vi "Rapid Read.vi"(0 "AlazarCluster":T10, 2 "Forward?":bool, 5 "Motion Settings":T2={"No Motion?"=FALSE, "Motion System"=enum."NI 735x", "Motion Bd ID"=1, "Motion Profile"="SMAC1", "# Axis"=1, "Reverse Z axis?"=TRUE, "SMAC Axis"=0, "scan pair"=enum."y-(x) scan", "RT fps"=6.0, "Steps per mm"=[1000, 1000, 1000, 1000], "Motor Parameters"={"velocity ct/s"=[10000.0, 10000.0, 10000.0, 50000.0], "accel ct/s^2"=[50000.0, 50000.0, 50000.0, 200000.0]}, "One Way Scan"=FALSE, "Reverse One Way Scan"=FALSE, "Global Position (mm)"=[], "Plane"=0, "Distance between\nscan lines (um)"=0.0, "Distance between\nscan planes (um)"=0.0, "number of scan planes"=1, "Total steps in line"=0, "Xtra plane\ndistance  (um)"=100, "Xtra planes "=1, "Add Axis"=FALSE, "overshoot cts"=200, "BKPT Shift"=0, "Scan Start Time (ms)"=0, "ESP VISA"="GPIB::1::INSTR", "3rd Axis"=1, "GL Ref Out"=refnum, "Galil Address"=""} {"3rd Axis" items=["x", "y", "z", "w"]; "Xtra planes" min=1; "Xtra plane\ndistance  (um)" min=0; "Distance between\nscan planes (um)" format="%.2f"; "Distance between\nscan lines (um)" format="%.2f"; "SMAC Axis" items=["None"=0, "Axis 1"=1, "Axis 2"=2, "Axis 3"=3, "Axis 4"=4, "Axis 5"=5, "Axis 6"=6, "Axis 7"=7, "Axis 8"=8, "Vector Space 1"=17, "Vector Space 2"=18, "Vector Space 3"=19, "Vector Space 4"=20]; "Motion Bd ID" min=1 max=32 step=1}, 7 "Digitizer Settings":T6={"Digitizer delay (us) "=0.0, "rf points per line"=2048, "lines per plane"=128, "Samp Rate (Hz)"=100000000.0, "Additional dig delay (us)"=0.0, "Voltage Scale"=0.4, "Pre-Looks"=0, "Offset delay (us)"=0.0, "bits A/D"=8, "Avg Num"=1, "DigTimeOut"=5.0, "Rel Dig Delay"=0.0, "Dig Ch"=0, "LeCroyCluster"={"LeCroy Channels"=[TRUE, FALSE, FALSE, FALSE], "LC read pt offset"=0.0, "Sweep Avg"=FALSE}, "Main Digitizer"=enum."NI Digitizer", "Dig Config"=enum."Single channel", "Digitizer ID Cluster"={"Acqiris/Alazar/SP ID"=[], "NI Instr Handles"=[], "LeCroy VISA"="", "GaGe Handle"={"Handle"=0, "Sample size"=0, "Resolution"=0, "Offset"=0, "Channels"=0, "Boards"=0}, "ATS Ref"="ATS9350", "Acqiris Address"=["PCI::INSTR0"], "ADQRef"=refnum, "adq_cu_ptr"=refnum}, "Trigger Settings"={"Trig Source"=1, "Trig Coupling"=0, "Trig Slope"=0, "Level (mV)"=1500.0}, "Bulk Acq"=FALSE, "Bulk Start Indexes"=[], "Data Ref RF"=refnum, "NI ID/Channel"=[], "Total Dig CH"=1, "Xtra Ann Trig delay (us)"=10.0, "Fix Z Delay?"=FALSE, "One Way Transmission?"=FALSE, "Data Ref Log"=refnum} {"Trigger Settings"."Trig Slope" items=["Positive", "Negative"]; "Trigger Settings"."Level (mV)" format="%.2f"; "Trigger Settings"."Trig Coupling" items=["DC 1 MOhm", "AC 1 MOhm", "DC 50 Ohm", "AC 50 Ohm"]; "Trigger Settings"."Trig Source" items=["Chan 1", "External"]; "Rel Dig Delay" format="%.2f"; "DigTimeOut" format="%.2f"; "Avg Num" min=1; "Offset delay (us)" format="%.2f"; "Additional dig delay (us)" format="%.2f"; "Digitizer delay (us)" format="%.2f"}, 9 "Location":T1=enum."WCM Main", 11 "error in":errorcluster, 12 "Pause?":bool, 13 "DigTimeOut":sgl=5.0 format="%.2f") -> (1 "gain":dbl, 4 "Array":i16[][](array[numeric]), 6 "Reverse?":bool, 8 "dig error":bool, 14 "gain 2 Ch":dbl, 15 "error out":errorcluster)   [LabVIEW 2022 SP3]
uses:
  -DigitizerRoutines/DigitizerSettings.ctl
  -DigitizerRoutines/Digitizer.ctl
  -DigitizerRoutines/DigConfig.ctl
  -DigitizerRoutines/DigitizerID.ctl
  C:/Windows/System32/ADQAPI_dotNet_helper.dll
  Windows/System32/ADQAPI_dotNet_helper.dll
  Motion Controllers/NI_controller/-NI_MotionRoutines/MotionParameters.ctl
  Motion Controllers/NI_controller/-NI_MotionRoutines/MotionSys.ctl
  Motion Controllers/-MotionRoutines/ScanAxis.ctl
  Motion Controllers/-MotionRoutines/3rdAxis.ctl
  -ScanSystem/Controls/location.ctl
  Motion Controllers/Galil/Command Menu.ctl
  <vilib>/DAQmx/write.llb/DAQmx Write (Digital Bool 1Line 1Point).vi
  Motion Controllers/-MotionRoutines/MotionGlobals.vi
  <vilib>/DAQmx/miscellaneous.llb/DAQmx Fill In Error Info.vi
  <instrlib>/niScope/Acquire/Fetch/niScope Multi Fetch Binary 8.vi
  <instrlib>/Acqiris Dx/Acqiris Dx.lvlib
  <vilib>/Motion/FlexMotion/CustomControls/CustomControls.llb/Program.flx
  <instrlib>/LeCroy Wave Series/LeCroy Wave Series.lvlib
panel:
  in  "Motion Program":u8=1 format="%.0x"
  # "1-D and 2-D B scan settings"
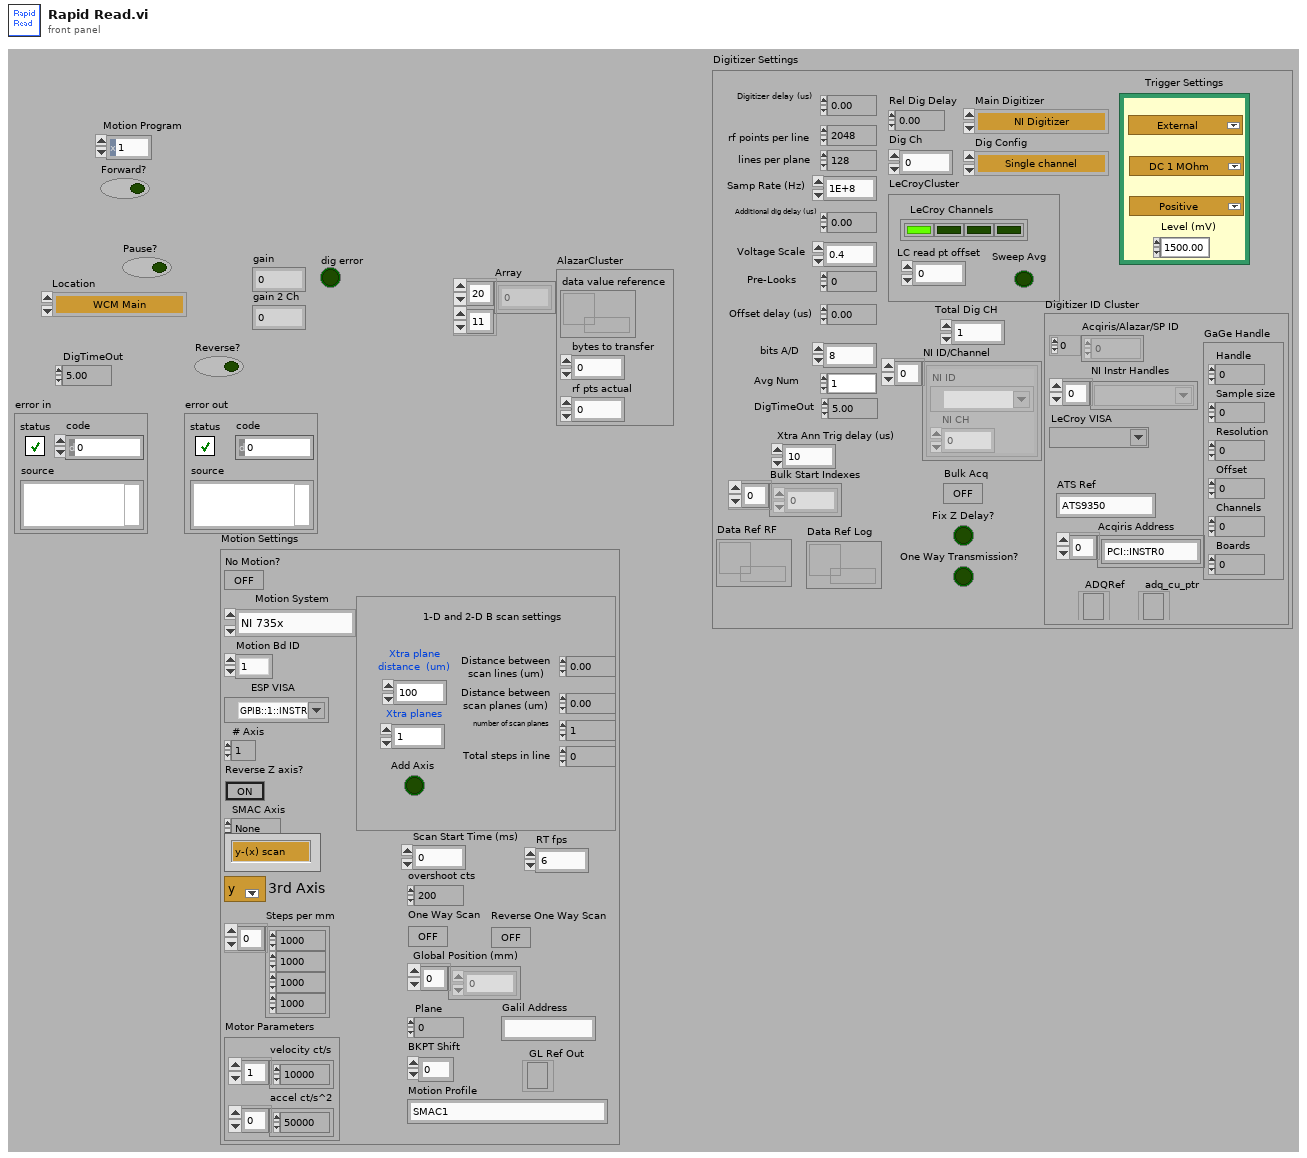
[diagram p1: front panel]
types:
  T1 = typedef "location.ctl" = enum16{"Automatic", "WCM Main", "Hawaii", "Columbia MM3000", "Columbia  NI System", "NYU", "RRI 2", "UHI Allen", "CUMC RT", "Chiba", "Stony Brook", "WCM Microscopy", "WCM Aeoretch", "WCM Optics Lab", "WCM Main 2Axis", "WCM Rotation", "WCM SAM SMAC", "SERI GP"}
  T2 = typedef "MotionParameters.ctl" = cluster{"No Motion?":bool, "Motion System":T3, "Motion Bd ID":u8, "Motion Profile":string, "# Axis":i8, "Reverse Z axis?":bool, "SMAC Axis":u16, "scan pair":T4, "RT fps":sgl, "Steps per mm":i32[], "Motor Parameters":cluster{"velocity ct/s":dbl[], "accel ct/s^2":dbl[]}, "One Way Scan":bool, "Reverse One Way Scan":bool, "Global Position (mm)":dbl[], "Plane":i32, "Distance between\nscan lines (um)":sgl, "Distance between\nscan planes (um)":sgl, "number of scan planes":i32, "Total steps in line":i32, "Xtra plane\ndistance  (um)":i32, "Xtra planes ":i32, "Add Axis":bool, "overshoot cts":i32, "BKPT Shift":i32, "Scan Start Time (ms)":u32, "ESP VISA":refnum<visa-resource-name>, "3rd Axis":T5, "GL Ref Out":refnum<k7>, "Galil Address":string}
  T3 = typedef "MotionSys.ctl" = enum16{"MM3000", "NI 735x", "Newport ESP", "No Motion Card", "Galil"}
  T4 = typedef "ScanAxis.ctl" = enum16{"y-(x) scan", "x-(y) scan", "z-(x) scan", "z-(y) scan", "y-(z) scan", "x-(z) scan", "w-(x) scan", "w-(y) scan", "w-(z) scan", "x-(w) scan", "y-(w) scan", "z-(w) scan"}
  T5 = typedef "3rdAxis.ctl" = u16
  T6 = typedef "DigitizerSettings.ctl" = cluster{"Digitizer delay (us) ":dbl, "rf points per line":i32, "lines per plane":i32, "Samp Rate (Hz)":dbl, "Additional dig delay (us)":dbl, "Voltage Scale":dbl, "Pre-Looks":i32, "Offset delay (us)":dbl, "bits A/D":i8, "Avg Num":i32, "DigTimeOut":sgl, "Rel Dig Delay":sgl, "Dig Ch":i32, "LeCroyCluster":cluster{"LeCroy Channels":bool[], "LC read pt offset":dbl, "Sweep Avg":bool}, "Main Digitizer":T7, "Dig Config":T8, "Digitizer ID Cluster":T9, "Trigger Settings":cluster{"Trig Source":u16, "Trig Coupling":u16, "Trig Slope":u16, "Level (mV)":dbl}, "Bulk Acq":bool, "Bulk Start Indexes":i32[], "Data Ref RF":refnum<data-value>, "NI ID/Channel":cluster{"NI ID":refnum<k15>, "NI CH":i32}[], "Total Dig CH":i32, "Xtra Ann Trig delay (us)":dbl, "Fix Z Delay?":bool, "One Way Transmission?":bool, "Data Ref Log":refnum<data-value>}
  T7 = typedef "Digitizer.ctl" = enum16{"Acqiris Digitizer", "NI Digitizer", "LeCroy", "GaGe", "AlazarTech", "No Digitizer", "Teledyne"}
  T8 = typedef "DigConfig.ctl" = enum16{"Single channel", "2 Chans w/ 2 Acqiris", "2 Chans w/ 1 Acqiris", "5-CH Pulser New", "5-CH pulser w/ ann array", "5-pass style ann array", "Empty"}
  T9 = typedef "DigitizerID.ctl" = cluster{"Acqiris/Alazar/SP ID":u32[], "NI Instr Handles":refnum<k15>[], "LeCroy VISA":refnum<visa-resource-name>, "GaGe Handle":cluster{"Handle":u32, "Sample size":u32, "Resolution":i32, "Offset":i32, "Channels":u32, "Boards":u32}, "ATS Ref":string, "Acqiris Address":string[], "ADQRef":refnum<k24>, "adq_cu_ptr":refnum<k24>}
  T10 = cluster{"data value reference":refnum<data-value>, "bytes to transfer":u32, "rf pts actual":u32}
  T11 = typedef "Command Menu.ctl" = enum16{"CommandPassThrough", "Abort Motion", "Define Pos", "Velocity", "Acceleration", "Deceleration", "Position Rel", "Postion Abs", "Begin Move", "After Move", "Home", "KI", "KD", "KP", "IL", "Config I/O", "Set Bit", "Clear Bit", "Motor Off", "Moto On", "Status", "Execute", "Halt Execute", "HX Status", "Tell Velocity", "Check Motion", "BreakPoint", "Tell Position", "Current Code Line", "Tell Switches", "OC Force On", "OC Off", "Pos Soft Limit", "Rev Soft Limit"}
  T12 = typedef "Program.flx" = u8
  T13 = typedef "Var" = u8
  T14 = typedef "Resource Out.flx" = u8
  T15 = cluster{"returnedSamplesPerSeg":i32, "indexFirstPoint":i32, "sampTime":dbl, "vGain":dbl, "vOffset":dbl, "returnedSegments":i32, "nbrAvgWforms":i32, "actualTriggersInAcqLo":u32, "actualTriggersInAcqHi":u32, "reserved3":dbl, "actualDataSize":u32, "missingValue":dbl}
  T16 = cluster{"actualSamples":i32, "absoluteInitialX":dbl, "relativeInitialX":dbl, "xIncrement":dbl, "offset":dbl, "gain":dbl, "reserved1":dbl, "reserved2":dbl}[]
  T17 = cluster{"actualSamples":i32, "absoluteInitialX":dbl, "relativeInitialX":dbl, "xIncrement":dbl, "offset":dbl, "gain":dbl, "reserved1":dbl, "reserved2":dbl}
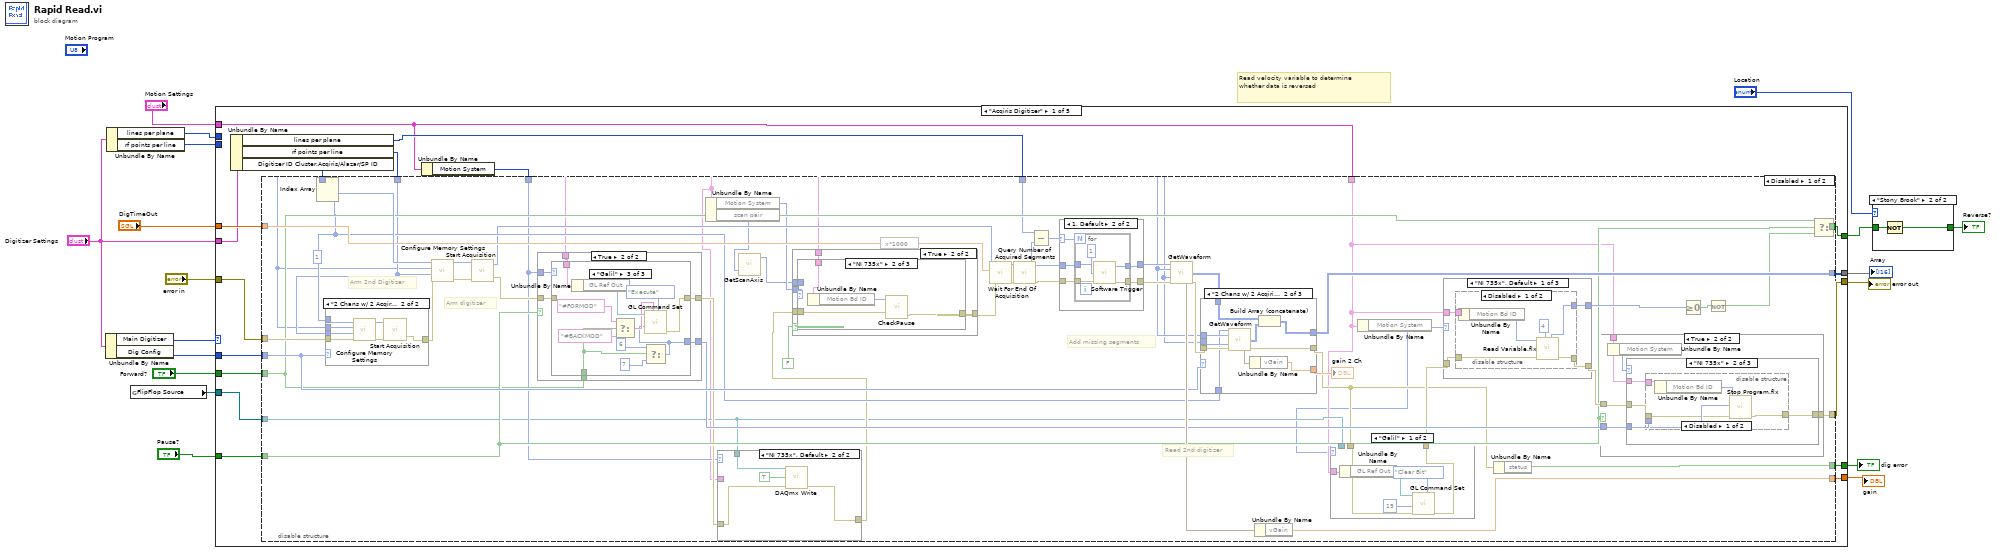
[diagram p0: block diagram]
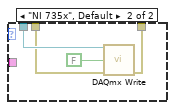
[diagram p3: hidden frame]
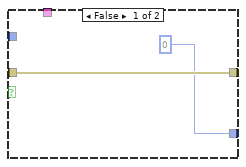
[diagram p4: hidden frame]
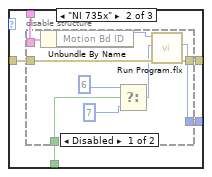
[diagram p6: hidden frame]
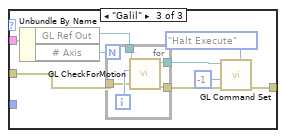
[diagram p11: hidden frame]
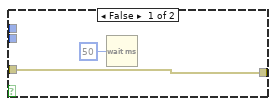
[diagram p12: hidden frame]
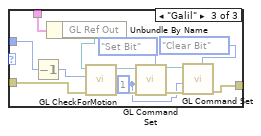
[diagram p14: hidden frame]
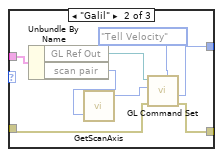
[diagram p16: hidden frame]
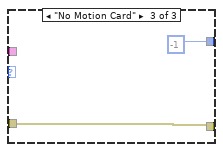
[diagram p17: hidden frame]
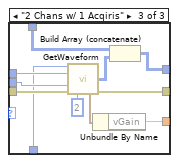
[diagram p19: hidden frame]
diagram:
  # "Read velocity variable to determine whether data is reversed"
  n1 = Unbundle By Name("Digitizer Settings") -> ("Main Digitizer"=w11:T7, "Dig Config"=w10:T8)
  n2 = Unbundle By Name("Digitizer Settings") -> ("lines per plane"=w8:i32, "rf points per line"=w7:i32)
  n3 = global read "MotionGlobals.vi" "FlipFlop Source"() -> (w14:refnum<k21>)
  n4 = case shown="\"Acqiris Digitizer\"" w11 {
    tunnel: [w26 w289 w441 w619 w763] -> w18
    tunnel: "error in" -> [w27 w284 w467 w614 w766]
    tunnel: w7 -> [_ _ _ _ _]
    tunnel: w8 -> [_ _ _ _ _]
    tunnel: [w35 w279 w459 w609 w789] -> w16
    tunnel: [w28 w295 w451 w626 w776] -> w5
    tunnel: "DigTimeOut" -> [w31 _ w458 _ w774]
    tunnel: [w34 w276 w461 w607 w785] -> w15
    tunnel: w14 -> [w20 w263 w432 w601 w762]
    tunnel: [w32 w297 w455 w629 w782] -> w13
    tunnel: "Digitizer Settings" -> [w30 w273 w445 w613 w768]
    tunnel: w10 -> [w29 _ _ _ _]
    tunnel: "Motion Settings" -> [w19 w259 w429 w599 w760]
    tunnel: "Pause?" -> [w25 w290 w442 w620 w773]
    tunnel: "Forward?" -> [w24 w291 w446 w622 _]
    frame "Acqiris Digitizer" {
      n5 = Unbundle By Name(w30) -> ("lines per plane"=w22:i32, "rf points per line"=w23:i32, "Digitizer ID Cluster.Acqiris/Alazar/SP ID"=w33:u32[])
      n6 = Unbundle By Name(w19) -> ("Motion System"=w21:T3)
      n7 = disable-structure shown="Disabled" {
        disable-tunnel: [w73 _] -> w35
        disable-tunnel: [w70 _] -> w34
        disable-tunnel: w33 -> [w67 _]
        disable-tunnel: [w66 _] -> w32
        disable-tunnel: w31 -> [w65 _]
        disable-tunnel: w29 -> [w63 _]
        disable-tunnel: [w61 _] -> w28
        disable-tunnel: w27 -> [w60 _]
        disable-tunnel: [w55 _] -> w26
        disable-tunnel: w25 -> [w53 _]
        disable-tunnel: w24 -> [w52 _]
        disable-tunnel: w23 -> [w45 _]
        disable-tunnel: w22 -> [w44 _]
        disable-tunnel: w21 -> [w41 _]
        disable-tunnel: w20 -> [w40 _]
        disable-tunnel: w19 -> [w37 _]
        frame Disabled {
          (unwired) 1 ("index")
          # "Read 2nd digitizer"
          # "Arm 2nd Digitizer"
          # "Arm digitizer"
          # "Add missing segments"
          n8 = Index Array(array=w67) -> (element #1=w68:u32, element #2=w50:u32)  [unwired: 2 in]
          n9 = case shown="\"2 Chans w/ 2 Acqiris\"" w63 {
            tunnel: w45 -> [_ w234]
            tunnel: w44 -> [_ w233]
            tunnel: w50 -> [_ w232]
            tunnel: w60 -> [w229 w231]
            tunnel: [w229 w230] -> w75
            frame "Single channel", Default {
            }
            frame "2 Chans w/ 2 Acqiris" {
              n10 = call <instrlib>:"Configure Memory Settings.vi"("error in (no error)"=w231, "Number of Samples (1000)"=w234, "Number of Segments (1)"=w233, "Instrument ID"=w232) -> ("error out"=w235:errorcluster, "dup Instrument ID"=w236:u32)  [unwired: 2 out]
              n11 = call <instrlib>:"Start Acquisition.vi"("error in (no error)"=w235, "Instrument ID"=w236) -> ("error out"=w230:errorcluster)  [unwired: 2 in, 1 out]
            }
          }
          n12 = call <instrlib>:"Configure Memory Settings.vi"("error in (no error)"=w75, "Number of Samples (1000)"=w45, "Number of Segments (1)"=w44, "Instrument ID"=w68) -> ("error out"=w78:errorcluster, "dup Instrument ID"=w79:u32)  [unwired: 2 out]
          n13 = call <instrlib>:"Start Acquisition.vi"("error in (no error)"=w78, "Instrument ID"=w79) -> ("error out"=w59:errorcluster, "dup Instrument ID"=w49:u32)  [unwired: 2 in]
          n14 = case shown="True" w53 {
            tunnel: w59 -> [w98 w104]
            tunnel: [w98 w103] -> w42
            tunnel: w52 -> [_ w102]
            tunnel: [u8 0 ("Resource Out") w101] -> w57
            tunnel: w41 -> [_ w100]
            tunnel: w37 -> [_ w99]
            frame False {
            }
            frame True {
              n15 = case shown="\"Galil\"" w100 {
                tunnel: w104 -> [w105 w110 _]
                tunnel: [w105 w109 w126] -> w103
                tunnel: w102 -> [_ w108 w122]
                tunnel: [_ w107 w120] -> w101
                tunnel: w99 -> [_ w106 w129]
                frame "MM3000", Default {
                }
                frame "NI 735x" {
                  n16 = disable-structure shown="Disabled" {
                    disable-tunnel: w110 -> [w119 _]
                    disable-tunnel: [w118 _] -> w109
                    disable-tunnel: w108 -> [w114 _]
                    disable-tunnel: [w113 _] -> w107
                    disable-tunnel: w106 -> [w112 _]
                    frame Disabled {
                      n17 = Unbundle By Name(w112) -> ("Motion Bd ID"=w111:u8)
                      n18 = Select(t=T12 6 ("Motion Program"), s=w114, f=T12 7 ("Motion Program")) -> (s? t:f=w115:T12)
                      n19 = call <vilib>:"Run Program.flx"("error in (no error)"=w119, "Program (1)"=w115, "Board ID"=w111) -> ("error out"=w118:errorcluster, "Resource Out"=w113:T14)  [unwired: 3 in, 1 out]
                    }
                    frame Enabled {
                    }
                  }
                }
                frame "Galil" {
                  n20 = Unbundle By Name(w129) -> ("GL Ref Out"=w128:refnum<k7>)
                  n21 = Select(t="#FORMOD" ("Program Name"), s=w122, f="#BACKMOD" ("Program Name")) -> (s? t:f=w127:string)
                  n22 = Select(t=u8 6 ("Motion Program"), s=w122, f=u8 7 ("Motion Program")) -> (s? t:f=w120:u8)
                  n23 = call "GL Command Set.vi"("Command"=Command_Menu."Execute", "Text Input"=w127, "Value"=w120, "Galil.IGalil"=w128) -> ("error out"=w126:errorcluster)  [unwired: 3 in, 4 out]
                }
              }
            }
          }
          n24 = Unbundle By Name(w37) -> ("Motion System"=w48:T3, "scan pair"=w47:T4)
          n25 = case shown="\"NI 735x\", Default" w41 {
            tunnel: w40 -> [_ w257]
            tunnel: w37 -> [w251 _]
            tunnel: w42 -> [w250 w256]
            tunnel: [w249 w255] -> w43
            frame "Galil" {
              n26 = Unbundle By Name(w251) -> ("GL Ref Out"=w254:refnum<k7>)
              n27 = call "GL Command Set.vi"("Command"=Command_Menu."Set Bit", "error in (no error)"=w250, "Value"=19, "Galil.IGalil"=w254) -> ("error out"=w249:errorcluster)  [unwired: 3 in, 4 out]
            }
            frame "NI 735x", Default {
              n28 = call-poly <vilib>:"DAQmx Write.vi"("task/channels in"=w257, "data"=TRUE ("stop (T)"), "error in"=w256) -> ("error out"=w255:errorcluster)  [unwired: 10 in, 2 out]
            }
          }
          n29 = call "GetScanAxis.vi"("scan pair"=w47) -> ("Axis 1"=w46:i32)  [unwired: 1 in, 2 out]
          n30 = case shown="True" FALSE {
            tunnel: w43 -> [w162 w167]
            tunnel: [w162 w166] -> w62
            tunnel: w37 -> [_ w165]
            tunnel: w48 -> [_ w164]
            tunnel: w46 -> [_ w163]
            frame False {
              n31 = Wait (ms)(milliseconds to wait=u32 50) -> ()  [unwired: 1 out]
            }
            frame True {
              n32 = case shown="\"NI 735x\"" w164 {
                tunnel: w167 -> [w168 w172 w179]
                tunnel: [w168 w171 w180] -> w166
                tunnel: w165 -> [_ w170 w178]
                tunnel: w163 -> [_ _ w176]
                frame "MM3000", Default {
                }
                frame "NI 735x" {
                  n33 = Unbundle By Name(w170) -> ("Motion Bd ID"=w169:u8)
                  n34 = call "CheckPause.vi"("error in"=w172, "Motion Board ID"=w169) -> ("error out"=w171:errorcluster)  [unwired: 3 in]
                }
                frame "Galil" {
                  w173 = 1 ("Value")
                  n35 = Decrement(x=w176) -> (x-1=w175:i32)
                  n36 = Unbundle By Name(w178) -> ("GL Ref Out"=w177:refnum<k7>)
                  n37 = call "GL CheckForMotion.vi"("error in"=w179, "Axis"=w175, "Refnum in"=w177) -> ("error out"=w184:errorcluster, "Refnum out"=w185:refnum<k7>)  [unwired: 6 in, 1 out]
                  n38 = call "GL Command Set.vi"("Command"=Command_Menu."Set Bit", "error in (no error)"=w184, "Value"=w173, "Galil.IGalil"=w185) -> ("error out"=w182:errorcluster, "ref out"=w181:refnum<k7>)  [unwired: 3 in, 3 out]
                  n39 = call "GL Command Set.vi"("Command"=Command_Menu."Clear Bit", "error in (no error)"=w182, "Value"=w173, "Galil.IGalil"=w181) -> ("error out"=w180:errorcluster)  [unwired: 3 in, 4 out]
                }
              }
            }
          }
          n40 = expression code="x*1000"(w65) -> (w64:sgl)
          n41 = call <instrlib>:"Wait For End Of Acquisition.vi"("error in (no error)"=w62, "Timeout"=w64, "Instrument ID"=w49) -> ("error out"=w77:errorcluster, "dup Instrument ID"=w83:u32)  [unwired: 3 out]
          n42 = call <instrlib>:"Query Number of Acquired Segments.vi"("error in (no error)"=w77, "Instrument ID"=w83) -> ("error out"=w85:errorcluster, "Number of Segments"=w86:i32, "dup Instrument ID"=w82:u32)  [unwired: 3 out]
          n43 = Subtract(x=w44, y=w86) -> (x-y=w81:i32)
          n44 = case shown="1, Default" w81 {
            selector: w81 -> [_ w239]
            tunnel: w85 -> [w237 w243]
            tunnel: [w237 w242] -> w84
            tunnel: w82 -> [w238 w241]
            tunnel: [w238 w240] -> w80
            frame 0 {
            }
            frame 1, Default {
              n45 = for {
                N: w239 -> [_]
                tunnel: w243 -> [w248]
                tunnel: w241 -> [w245]
                tunnel: [w247] -> w242
                tunnel: [w244] -> w240
                n46 = call <instrlib>:"Software Trigger.vi"("error in (no error)"=w248, "Type"=1, "Instrument ID"=w245) -> ("error out"=w247:errorcluster, "dup Instrument ID"=w244:u32)
              }
            }
          }
          n47 = call "GetWaveform.vi"("Acq ID Out"=w80, "Num Samps"=w45, "Num Segs"=w44, "error in"=w84) -> ("Acquired Waveform16 bit"=w72:i16[][], "dataDesc"=w71:T15, "error out"=w74:errorcluster)  [unwired: 2 in, 7 out]
          n48 = case shown="\"2 Chans w/ 2 Acqiris\"" w63 {
            tunnel: w74 -> [w207 w217 w228]
            tunnel: [w207 w216 w227] -> w38
            tunnel: w44 -> [_ w215 w226]
            tunnel: w45 -> [_ w214 w225]
            tunnel: w50 -> [_ w213 w224]
            tunnel: [w206 w210 w221] -> w73
            tunnel: w72 -> [w206 w212 w223]
            tunnel: [_ w208 w218] -> w69
            frame "Single channel", Default {
            }
            frame "2 Chans w/ 2 Acqiris" {
              n49 = call "GetWaveform.vi"("Acq ID Out"=w213, "Num Samps"=w214, "Num Segs"=w215, "error in"=w217) -> ("Acquired Waveform16 bit"=w211:i16[][], "dataDesc"=w209:T15, "error out"=w216:errorcluster)  [unwired: 2 in, 7 out]
              n50 = Unbundle By Name(w209) -> ("vGain"=w208:dbl)
              n51 = Build Array (concatenate)(w212, w211) -> (w210:i16[][])
            }
            frame "2 Chans w/ 1 Acqiris" {
              n52 = call "GetWaveform.vi"("Acq ID Out"=w224, "Num Samps"=w225, "Num Segs"=w226, "error in"=w228, "Channel"=2) -> ("Acquired Waveform16 bit"=w222:i16[][], "dataDesc"=w219:T15, "error out"=w227:errorcluster)  [unwired: 1 in, 7 out]
              n53 = Unbundle By Name(w219) -> ("vGain"=w218:dbl)
              n54 = Build Array (concatenate)(w223, w222) -> (w221:i16[][])
            }
          }
          "gain 2 Ch" <- w69
          n55 = Unbundle By Name(w71) -> ("vGain"=w70:dbl)
          n56 = Unbundle By Name(w37) -> ("Motion System"=w36:T3)
          n57 = case shown="\"Galil\"" w36 {
            tunnel: w40 -> [_ w95]
            tunnel: w37 -> [w89 _]
            tunnel: w38 -> [w88 w94]
            tunnel: [w87 w93] -> w39
            frame "Galil" {
              n58 = Unbundle By Name(w89) -> ("GL Ref Out"=w92:refnum<k7>)
              n59 = call "GL Command Set.vi"("Command"=Command_Menu."Clear Bit", "error in (no error)"=w88, "Value"=19, "Galil.IGalil"=w92) -> ("error out"=w87:errorcluster)  [unwired: 3 in, 4 out]
            }
            frame "NI 735x", Default {
              n60 = call-poly <vilib>:"DAQmx Write.vi"("task/channels in"=w95, "data"=FALSE ("stop (T)"), "error in"=w94) -> ("error out"=w93:errorcluster)  [unwired: 10 in, 2 out]
            }
          }
          n61 = case shown="\"NI 735x\", Default" w36 {
            tunnel: [w186 w197 -1 ("Output")] -> w76
            tunnel: [w189 w198 w204] -> w58
            tunnel: w39 -> [w188 w199 w204]
            tunnel: w37 -> [w187 w196 _]
            frame "NI 735x", Default {
              n62 = disable-structure shown="Disabled" {
                disable-tunnel: [w194 _] -> w189
                disable-tunnel: w188 -> [w193 _]
                disable-tunnel: w187 -> [w192 _]
                disable-tunnel: [w191 _] -> w186
                frame Disabled {
                  n63 = Unbundle By Name(w192) -> ("Motion Bd ID"=w190:u8)
                  n64 = call <vilib>:"Read Variable.flx"("Var"=T13 4, "error in (no error)"=w193, "Board ID"=w190) -> ("error out"=w194:errorcluster, "Output"=w191:i32)  [unwired: 1 in, 4 out]
                }
                frame Enabled {
                }
              }
            }
            frame "Galil" {
              n65 = Unbundle By Name(w196) -> ("GL Ref Out"=w202:refnum<k7>, "scan pair"=w201:T4)
              n66 = call "GetScanAxis.vi"("scan pair"=w201) -> ("Axis 1"=w200:i32)  [unwired: 1 in, 2 out]
              n67 = call "GL Command Set.vi"("Command"=Command_Menu."Tell Velocity", "error in (no error)"=w199, "Axis"=w200, "Galil.IGalil"=w202) -> ("error out"=w198:errorcluster, "Response#"=w197:i32)  [unwired: 3 in, 3 out]
            }
            frame "No Motion Card" {
            }
          }
          n68 = Unbundle By Name(w38) -> ("status"=w66:bool)
          n69 = case shown="True" w53 {
            tunnel: w57 -> [_ w135]
            tunnel: w58 -> [w131 w134]
            tunnel: [w131 w136] -> w55
            tunnel: w37 -> [_ w133]
            frame False {
            }
            frame True {
              n70 = Unbundle By Name(w133) -> ("Motion System"=w132:T3)
              n71 = case shown="\"NI 735x\"" w132 {
                tunnel: [w137 w141 w149] -> w136
                tunnel: w135 -> [_ w140 _]
                tunnel: w134 -> [w137 w138 w152]
                tunnel: w133 -> [_ w139 w153]
                frame "MM3000", Default {
                }
                frame "NI 735x" {
                  n72 = disable-structure shown="Disabled" {
                    disable-tunnel: [w146 _] -> w141
                    disable-tunnel: w140 -> [w145 _]
                    disable-tunnel: w139 -> [w143 _]
                    disable-tunnel: w138 -> [w142 _]
                    frame Disabled {
                      n73 = Unbundle By Name(w143) -> ("Motion Bd ID"=w144:u8)
                      n74 = call <vilib>:"Stop Program.flx"("error in (no error)"=w142, "Program (1)"=w145, "Board ID"=w144) -> ("error out"=w146:errorcluster)  [unwired: 3 in, 2 out]
                    }
                    frame Enabled {
                    }
                  }
                }
                frame "Galil" {
                  n75 = Unbundle By Name(w153) -> ("GL Ref Out"=w154:refnum<k7>, "# Axis"=w155:i8)
                  n76 = for {
                    N: w155 -> [_]
                    tunnel: [w160] -> w151
                    tunnel: w154 -> [w159]
                    tunnel: w152 -> [w157]
                    tunnel: [w156] -> w150
                    i -> [w158]
                    n77 = call "GL CheckForMotion.vi"("error in"=w157, "Axis"=w158, "Refnum in"=w159) -> ("error out"=w160:errorcluster, "Refnum out"=w156:refnum<k7>)  [unwired: 6 in, 1 out]
                  }
                  n78 = call "GL Command Set.vi"("Command"=Command_Menu."Halt Execute", "error in (no error)"=w151, "Value"=-1, "Galil.IGalil"=w150) -> ("error out"=w149:errorcluster)  [unwired: 3 in, 4 out]
                }
              }
            }
          }
          n79 = Greater Or Equal To 0?(x=w76) -> (x >= 0?=w54:bool)
          n80 = Not(x=w54) -> (.not. x?=w51:bool)
          n81 = Select(t=w52, s=w53, f=w51) -> (s? t:f=w61:bool)
        }
        frame Enabled {
        }
      }
    }
    frame "Teledyne" {
      # "Set flip flop to take next frame edge"
      # "Arm digitizer"
      n82 = Unbundle By Name(w273) -> ("Digitizer ID Cluster.ADQRef"=w283:refnum<k24>, "Digitizer ID Cluster.adq_cu_ptr"=w282:refnum<k24>, "Digitizer ID Cluster.GaGe Handle.Boards"=w281:u32)
      n83 = call "SPADQ_DisarmArmTrigger.vi"("error in (no error)"=w284, "adq_num"=w281, "adq_cu_ptr in"=w282, "ADQAPI Ref"=w283) -> ("error out"=w286:errorcluster, "ADQAPI Ref (out)"=w285:refnum<k24>)  [unwired: 6 in]
      n84 = call "SPADQ_ArmTrigger.vi"("error in (no error)"=w286, "adq_num"=w281, "adq_cu_ptr in"=w282, "ADQAPI Ref"=w285) -> ("error out"=w280:errorcluster)  [unwired: 6 in, 1 out]
      n85 = Unbundle By Name(w259) -> ("Motion System"=w266:T3)
      n86 = case shown="False" w290 {
        tunnel: w280 -> [w347 w353]
        tunnel: [w347 w352] -> w265
        tunnel: w291 -> [_ w351]
        tunnel: [u8 0 ("Resource Out") w350] -> w294
        tunnel: w266 -> [_ w349]
        tunnel: w259 -> [_ w348]
        frame False {
        }
        frame True {
          n87 = case shown="\"Galil\"" w349 {
            tunnel: w353 -> [w354 w359 _]
            tunnel: [w354 w358 w374] -> w352
            tunnel: w351 -> [_ w357 w370]
            tunnel: [_ w355 _] -> w350
            tunnel: w348 -> [_ w356 w373]
            frame "MM3000", Default {
            }
            frame "NI 735x" {
              n88 = disable-structure shown="Disabled" {
                disable-tunnel: w359 -> [w368 _]
                disable-tunnel: [w367 _] -> w358
                disable-tunnel: w357 -> [w363 _]
                disable-tunnel: w356 -> [w362 _]
                disable-tunnel: [w360 _] -> w355
                frame Disabled {
                  n89 = Unbundle By Name(w362) -> ("Motion Bd ID"=w361:u8)
                  n90 = Select(t=T12 6 ("Motion Program"), s=w363, f=T12 7 ("Motion Program")) -> (s? t:f=w364:T12)
                  n91 = call <vilib>:"Run Program.flx"("error in (no error)"=w368, "Program (1)"=w364, "Board ID"=w361) -> ("error out"=w367:errorcluster, "Resource Out"=w360:T14)  [unwired: 3 in, 1 out]
                }
                frame Enabled {
                }
              }
            }
            frame "Galil" {
              n92 = Unbundle By Name(w373) -> ("GL Ref Out"=w378:refnum<k7>)
              n93 = Select(t="#FORMOD" ("Program Name"), s=w370, f="#BACKMOD" ("Program Name")) -> (s? t:f=w377:string)
              n94 = Select(t=u8 6 ("Motion Program"), s=w370, f=u8 7 ("Motion Program")) -> (s? t:f=w371:u8)
              n95 = call "GL Command Set.vi"("Command"=Command_Menu."Execute", "Text Input"=w377, "Value"=w371, "Galil.IGalil"=w378) -> ("error out"=w374:errorcluster)  [unwired: 3 in, 4 out]
            }
          }
        }
      }
      n96 = case shown="\"NI 735x\", Default" w266 {
        tunnel: w263 -> [_ w316]
        tunnel: w265 -> [w310 w315]
        tunnel: [w309 w314] -> w264
        tunnel: w259 -> [w308 _]
        frame "Galil" {
          n97 = Unbundle By Name(w308) -> ("GL Ref Out"=w313:refnum<k7>)
          n98 = call "GL Command Set.vi"("Command"=Command_Menu."Set Bit", "error in (no error)"=w310, "Value"=19, "Galil.IGalil"=w313) -> ("error out"=w309:errorcluster)  [unwired: 3 in, 4 out]
        }
        frame "NI 735x", Default {
          n99 = call-poly <vilib>:"DAQmx Write.vi"("task/channels in"=w316, "data"=TRUE ("stop (T)"), "error in"=w315) -> ("error out"=w314:errorcluster)  [unwired: 10 in, 2 out]
        }
      }
      n100 = Unbundle By Name(w259) -> ("Motion System"=w260:T3)
      n101 = case shown="True" FALSE {
        tunnel: w264 -> [w381 w385]
        tunnel: [w381 w384] -> w287
        tunnel: w259 -> [_ w383]
        tunnel: w260 -> [_ w382]
        frame False {
          n102 = Wait (ms)(milliseconds to wait=u32 50) -> ()  [unwired: 1 out]
        }
        frame True {
          n103 = case shown="\"NI 735x\"" w382 {
            tunnel: w385 -> [w386 w390]
            tunnel: [w386 w389] -> w384
            tunnel: w383 -> [_ w388]
            frame "MM3000", Default {
            }
            frame "NI 735x" {
              n104 = Unbundle By Name(w388) -> ("Motion Bd ID"=w387:u8)
              n105 = call "CheckPause.vi"("error in"=w390, "Motion Board ID"=w387) -> ("error out"=w389:errorcluster)  [unwired: 3 in]
            }
          }
        }
      }
      n106 = case shown="\"NI 735x\", Default" w260 {
        tunnel: w287 -> [w411 w419 w427]
        tunnel: [w410 w419 w427] -> w274
        tunnel: [w409 -5 ("Output") w421] -> w288
        tunnel: w259 -> [w408 _ w426]
        frame "NI 735x", Default {
          n107 = disable-structure shown="Disabled" {
            disable-tunnel: w411 -> [w416 _]
            disable-tunnel: [w415 _] -> w410
            disable-tunnel: [w414 _] -> w409
            disable-tunnel: w408 -> [w413 _]
            frame Disabled {
              n108 = Unbundle By Name(w413) -> ("Motion Bd ID"=w412:u8)
              n109 = call <vilib>:"Read Variable.flx"("Var"=T13 4, "error in (no error)"=w416, "Board ID"=w412) -> ("error out"=w415:errorcluster, "Output"=w414:i32)  [unwired: 1 in, 4 out]
            }
            frame Enabled {
            }
          }
        }
        frame "No Motion Card" {
        }
        frame "Galil" {
          (unwired) -5 ("Output")
          n110 = Unbundle By Name(w426) -> ("GL Ref Out"=w425:refnum<k7>, "scan pair"=w423:T4)
          n111 = call "GetScanAxis.vi"("scan pair"=w423) -> ("Axis 1"=w422:i32)  [unwired: 1 in, 2 out]
          n112 = Decrement(x=w422) -> (x-1=w420:i32)
          n113 = call "GL Command Set.vi"("Command"=Command_Menu."Tell Velocity", "Axis"=w420, "Galil.IGalil"=w425) -> ("Response#"=w421:i32)  [unwired: 4 in, 4 out]
        }
      }
      n114 = Unbundle By Name(w273) -> ("Digitizer ID Cluster.ADQRef"=w272:refnum<k24>, "Digitizer ID Cluster.adq_cu_ptr"=w271:refnum<k24>, "Digitizer ID Cluster.GaGe Handle.Boards"=w270:u32, "DigTimeOut"=w269:sgl)
      n115 = Multiply(x=w269, y=sgl 1000.0) -> (x*y=w268:sgl)
      n116 = call "SPADQ_AcquisitionStatus.vi"("WaitTime (ms)"=w268, "error in (no error)"=w274, "adq_num"=w270, "adq_cu_ptr in"=w271, "ADQAPI Ref"=w272) -> ("error out"=w275:errorcluster)  [unwired: 3 in, 3 out]
      n117 = call "SPADQ_GetData.vi"("DelayCorrect?"=TRUE, "error in (no error)"=w275, "Digitizer Settings"=w273) -> ("error out"=w277:errorcluster, "Data Out"=w279:i16[][])  [unwired: 6 in, 1 out]
      n118 = case shown="\"NI 735x\", Default" w260 {
        tunnel: w277 -> [w393 w403 w407]
        tunnel: [w392 w402 w407] -> w262
        tunnel: w259 -> [w391 w405 _]
        frame "NI 735x", Default {
          n119 = disable-structure shown="Disabled" {
            disable-tunnel: w393 -> [w397 _]
            disable-tunnel: [w396 _] -> w392
            disable-tunnel: w391 -> [w395 _]
            frame Disabled {
              n120 = Unbundle By Name(w395) -> ("Motion Bd ID"=w394:u8)
              n121 = call <vilib>:"Read Variable.flx"("Var"=T13 4, "error in (no error)"=w397, "Board ID"=w394) -> ("error out"=w396:errorcluster)  [unwired: 1 in, 5 out]
            }
            frame Enabled {
            }
          }
        }
        frame "Galil" {
          n122 = Unbundle By Name(w405) -> ("GL Ref Out"=w404:refnum<k7>, "scan pair"=w401:T4)
          n123 = call "GetScanAxis.vi"("scan pair"=w401) -> ("Axis 1"=w400:i32)  [unwired: 1 in, 2 out]
          n124 = Decrement(x=w400) -> (x-1=w399:i32)
          n125 = call "GL Command Set.vi"("Command"=Command_Menu."Tell Velocity", "error in (no error)"=w403, "Axis"=w399, "Galil.IGalil"=w404) -> ("error out"=w402:errorcluster)  [unwired: 3 in, 4 out]
        }
        frame "No Motion Card" {
        }
      }
      n126 = call "Alazar_ConvertRaw.vi"("Digitizer Settings"=w273) -> ("Voltage multiplier"=w276:dbl)  [unwired: 9 in, 1 out]
      n127 = case shown="\"NI 735x\", Default" w260 {
        tunnel: w263 -> [_ w306]
        tunnel: w259 -> [w300 _]
        tunnel: w262 -> [w299 w305]
        tunnel: [w298 w304] -> w261
        frame "Galil" {
          n128 = Unbundle By Name(w300) -> ("GL Ref Out"=w303:refnum<k7>)
          n129 = call "GL Command Set.vi"("Command"=Command_Menu."Clear Bit", "error in (no error)"=w299, "Value"=19, "Galil.IGalil"=w303) -> ("error out"=w298:errorcluster)  [unwired: 3 in, 4 out]
        }
        frame "NI 735x", Default {
          n130 = call-poly <vilib>:"DAQmx Write.vi"("task/channels in"=w306, "data"=FALSE ("stop (T)"), "error in"=w305) -> ("error out"=w304:errorcluster)  [unwired: 10 in, 2 out]
        }
      }
      n131 = Less Than 0?(x=w288) -> (x < 0?=w296:bool)
      n132 = Not(x=w296) -> (.not. x?=w292:bool)
      n133 = case shown="False" w290 {
        tunnel: w294 -> [_ w323]
        tunnel: w261 -> [w318 w321]
        tunnel: [w318 w322] -> w289
        tunnel: w259 -> [_ w320]
        frame False {
        }
        frame True {
          n134 = Unbundle By Name(w320) -> ("Motion System"=w319:T3)
          n135 = case shown="\"NI 735x\"" w319 {
            tunnel: w323 -> [_ w328 _]
            tunnel: [w324 w327 w336] -> w322
            tunnel: w321 -> [w324 w326 w339]
            tunnel: w320 -> [_ w325 w341]
            frame "MM3000", Default {
            }
            frame "NI 735x" {
              n136 = disable-structure shown="Disabled" {
                disable-tunnel: w328 -> [w333 _]
                disable-tunnel: [w332 _] -> w327
                disable-tunnel: w326 -> [w331 _]
                disable-tunnel: w325 -> [w330 _]
                frame Disabled {
                  n137 = Unbundle By Name(w330) -> ("Motion Bd ID"=w329:u8)
                  n138 = call <vilib>:"Stop Program.flx"("error in (no error)"=w331, "Program (1)"=w333, "Board ID"=w329) -> ("error out"=w332:errorcluster)  [unwired: 3 in, 2 out]
                }
                frame Enabled {
                }
              }
            }
            frame "Galil" {
              n139 = Unbundle By Name(w341) -> ("GL Ref Out"=w335:refnum<k7>, "# Axis"=w340:i8)
              n140 = for {
                N: w340 -> [_]
                tunnel: [w345] -> w337
                tunnel: w335 -> [w344]
                tunnel: w339 -> [w342]
                i -> [w343]
                n141 = call "GL CheckForMotion.vi"("error in"=w342, "Axis"=w343, "Refnum in"=w344) -> ("error out"=w345:errorcluster)  [unwired: 6 in, 2 out]
              }
              n142 = call "GL Command Set.vi"("Command"=Command_Menu."Halt Execute", "error in (no error)"=w337, "Value"=-1, "Galil.IGalil"=w335) -> ("error out"=w336:errorcluster)  [unwired: 3 in, 4 out]
            }
          }
        }
      }
      n143 = Select(t=w292, s=w290, f=w291) -> (s? t:f=w295:bool)
      n144 = Unbundle By Name(w289) -> ("status"=w297:bool)
    }
    frame "NI Digitizer", Default {
      # "Set flip flop to take next frame edge"
      # "Arm digitizer"
      n145 = Unbundle By Name(w445) -> ("Digitizer ID Cluster.NI Instr Handles"=w457:refnum<k15>[])
      n146 = Index Array(array=w457) -> (element=w456:refnum<k15>)  [unwired: 1 in]
      n147 = call <instrlib>:"niScope Initiate Acquisition.vi"("instrument handle"=w456, "error in"=w467) -> ("instrument handle out"=w468:refnum<k15>, "error out"=w450:errorcluster)  [unwired: 1 in, 11 out]
      n148 = Unbundle By Name(w429) -> ("Motion System"=w444:T3)
      n149 = case shown="True" w442 {
        tunnel: w450 -> [w518 w524]
        tunnel: [w518 w523] -> w435
        tunnel: w446 -> [_ w522]
        tunnel: [u8 0 ("Resource Out") w521] -> w449
        tunnel: w444 -> [_ w520]
        tunnel: w429 -> [_ w519]
        frame False {
        }
        frame True {
          n150 = case shown="\"Galil\"" w520 {
            tunnel: w524 -> [w525 w530 _]
            tunnel: [w525 w529 w545] -> w523
            tunnel: w522 -> [_ w528 w541]
            tunnel: [_ w526 _] -> w521
            tunnel: w519 -> [_ w527 w544]
            frame "MM3000", Default {
            }
            frame "NI 735x" {
              n151 = disable-structure shown="Disabled" {
                disable-tunnel: w530 -> [w539 _]
                disable-tunnel: [w538 _] -> w529
                disable-tunnel: w528 -> [w534 _]
                disable-tunnel: w527 -> [w533 _]
                disable-tunnel: [w531 _] -> w526
                frame Disabled {
                  n152 = Unbundle By Name(w533) -> ("Motion Bd ID"=w532:u8)
                  n153 = Select(t=T12 6 ("Motion Program"), s=w534, f=T12 7 ("Motion Program")) -> (s? t:f=w535:T12)
                  n154 = call <vilib>:"Run Program.flx"("error in (no error)"=w539, "Program (1)"=w535, "Board ID"=w532) -> ("error out"=w538:errorcluster, "Resource Out"=w531:T14)  [unwired: 3 in, 1 out]
                }
                frame Enabled {
                }
              }
            }
            frame "Galil" {
              n155 = Unbundle By Name(w544) -> ("GL Ref Out"=w549:refnum<k7>)
              n156 = Select(t="#FORMOD" ("Program Name"), s=w541, f="#BACKMOD" ("Program Name")) -> (s? t:f=w548:string)
              n157 = Select(t=u8 6 ("Motion Program"), s=w541, f=u8 7 ("Motion Program")) -> (s? t:f=w542:u8)
              n158 = call "GL Command Set.vi"("Command"=Command_Menu."Execute", "Text Input"=w548, "Value"=w542, "Galil.IGalil"=w549) -> ("error out"=w545:errorcluster)  [unwired: 3 in, 4 out]
            }
          }
        }
      }
      n159 = Unbundle By Name(w429) -> ("Motion System"=w433:T3)
      n160 = case shown="\"NI 735x\", Default" w433 {
        tunnel: w432 -> [_ w487]
        tunnel: w429 -> [w481 _]
        tunnel: w435 -> [w480 w486]
        tunnel: [w479 w485] -> w434
        frame "Galil" {
          n161 = Unbundle By Name(w481) -> ("GL Ref Out"=w484:refnum<k7>)
          n162 = call "GL Command Set.vi"("Command"=Command_Menu."Set Bit", "error in (no error)"=w480, "Value"=19, "Galil.IGalil"=w484) -> ("error out"=w479:errorcluster)  [unwired: 3 in, 4 out]
        }
        frame "NI 735x", Default {
          n163 = call-poly <vilib>:"DAQmx Write.vi"("task/channels in"=w487, "data"=TRUE ("stop (T)"), "error in"=w486) -> ("error out"=w485:errorcluster)  [unwired: 10 in, 2 out]
        }
      }
      n164 = Unbundle By Name(w429) -> ("Motion System"=w443:T3)
      n165 = case shown="True" FALSE {
        tunnel: w434 -> [w552 w556]
        tunnel: [w552 w555] -> w439
        tunnel: w429 -> [_ w554]
        tunnel: w443 -> [_ w553]
        frame False {
          n166 = Wait (ms)(milliseconds to wait=u32 50) -> ()  [unwired: 1 out]
        }
        frame True {
          n167 = case shown="\"NI 735x\"" w553 {
            tunnel: w556 -> [w557 w561]
            tunnel: [w557 w560] -> w555
            tunnel: w554 -> [_ w559]
            frame "MM3000", Default {
            }
            frame "NI 735x" {
              n168 = Unbundle By Name(w559) -> ("Motion Bd ID"=w558:u8)
              n169 = call "CheckPause.vi"("error in"=w561, "Motion Board ID"=w558) -> ("error out"=w560:errorcluster)  [unwired: 3 in]
            }
          }
        }
      }
      n170 = Unbundle By Name(w445) -> ("rf points per line"=w436:i32, "Dig Ch"=w454:i32)
      n171 = case shown="\"NI 735x\", Default" w443 {
        tunnel: w439 -> [w582 w590 w598]
        tunnel: [w581 w590 w598] -> w438
        tunnel: [w580 -5 ("Output") w592] -> w440
        tunnel: w429 -> [w579 _ w597]
        frame "NI 735x", Default {
          n172 = disable-structure shown="Disabled" {
            disable-tunnel: w582 -> [w587 _]
            disable-tunnel: [w586 _] -> w581
            disable-tunnel: [w585 _] -> w580
            disable-tunnel: w579 -> [w584 _]
            frame Disabled {
              n173 = Unbundle By Name(w584) -> ("Motion Bd ID"=w583:u8)
              n174 = call <vilib>:"Read Variable.flx"("Var"=T13 4, "error in (no error)"=w587, "Board ID"=w583) -> ("error out"=w586:errorcluster, "Output"=w585:i32)  [unwired: 1 in, 4 out]
            }
            frame Enabled {
            }
          }
        }
        frame "No Motion Card" {
        }
        frame "Galil" {
          (unwired) -5 ("Output")
          n175 = Unbundle By Name(w597) -> ("GL Ref Out"=w596:refnum<k7>, "scan pair"=w594:T4)
          n176 = call "GetScanAxis.vi"("scan pair"=w594) -> ("Axis 1"=w593:i32)  [unwired: 1 in, 2 out]
          n177 = Decrement(x=w593) -> (x-1=w591:i32)
          n178 = call "GL Command Set.vi"("Command"=Command_Menu."Tell Velocity", "Axis"=w591, "Galil.IGalil"=w596) -> ("Response#"=w592:i32)  [unwired: 4 in, 4 out]
        }
      }
      n179 = Number To Decimal String(number=w454) -> (decimal integer string=w453:string)  [unwired: 1 in]
      n180 = property class="niScope"(reference=w468, error in=w438, "Fetch Record Number"=0, "Fetch Number of Records"=-1) -> (reference out=w464:refnum<k15>, error out=w437:errorcluster)
      n181 = call-poly <instrlib>:"niScope Fetch (poly).vi"("timeout"=w458, "error in"=w437, "numSamples"=w436, "channels"=w453, "instrument handle"=w464) -> ("error out"=w460:errorcluster, "wfm"=w459:i8[][], "wfm info"=w463:T16)  [unwired: 4 out]
      n182 = case shown="\"NI 735x\", Default" w443 {
        tunnel: w460 -> [w564 w574 w578]
        tunnel: [w563 w573 w578] -> w431
        tunnel: w429 -> [w562 w576 _]
        frame "NI 735x", Default {
          n183 = disable-structure shown="Disabled" {
            disable-tunnel: w564 -> [w568 _]
            disable-tunnel: [w567 _] -> w563
            disable-tunnel: w562 -> [w566 _]
            frame Disabled {
              n184 = Unbundle By Name(w566) -> ("Motion Bd ID"=w565:u8)
              n185 = call <vilib>:"Read Variable.flx"("Var"=T13 4, "error in (no error)"=w568, "Board ID"=w565) -> ("error out"=w567:errorcluster)  [unwired: 1 in, 5 out]
            }
            frame Enabled {
            }
          }
        }
        frame "Galil" {
          n186 = Unbundle By Name(w576) -> ("GL Ref Out"=w575:refnum<k7>, "scan pair"=w572:T4)
          n187 = call "GetScanAxis.vi"("scan pair"=w572) -> ("Axis 1"=w571:i32)  [unwired: 1 in, 2 out]
          n188 = Decrement(x=w571) -> (x-1=w570:i32)
          n189 = call "GL Command Set.vi"("Command"=Command_Menu."Tell Velocity", "error in (no error)"=w574, "Axis"=w570, "Galil.IGalil"=w575) -> ("error out"=w573:errorcluster)  [unwired: 3 in, 4 out]
        }
        frame "No Motion Card" {
        }
      }
      n190 = Unbundle By Name(w429) -> ("Motion System"=w428:T3)
      n191 = case shown="\"NI 735x\", Default" w428 {
        tunnel: w432 -> [_ w477]
        tunnel: w429 -> [w471 _]
        tunnel: w431 -> [w470 w476]
        tunnel: [w469 w475] -> w430
        frame "Galil" {
          n192 = Unbundle By Name(w471) -> ("GL Ref Out"=w474:refnum<k7>)
          n193 = call "GL Command Set.vi"("Command"=Command_Menu."Clear Bit", "error in (no error)"=w470, "Value"=19, "Galil.IGalil"=w474) -> ("error out"=w469:errorcluster)  [unwired: 3 in, 4 out]
        }
        frame "NI 735x", Default {
          n194 = call-poly <vilib>:"DAQmx Write.vi"("task/channels in"=w477, "data"=FALSE ("stop (T)"), "error in"=w476) -> ("error out"=w475:errorcluster)  [unwired: 10 in, 2 out]
        }
      }
      n195 = Less Than 0?(x=w440) -> (x < 0?=w452:bool)
      n196 = Not(x=w452) -> (.not. x?=w447:bool)
      n197 = Select(t=w447, s=w442, f=w446) -> (s? t:f=w451:bool)
      n198 = case shown="True" w442 {
        tunnel: w449 -> [_ w494]
        tunnel: w430 -> [w489 w492]
        tunnel: [w489 w493] -> w441
        tunnel: w429 -> [_ w491]
        frame False {
        }
        frame True {
          n199 = Unbundle By Name(w491) -> ("Motion System"=w490:T3)
          n200 = case shown="\"NI 735x\"" w490 {
            tunnel: w494 -> [_ w499 _]
            tunnel: [w495 w498 w507] -> w493
            tunnel: w492 -> [w495 w497 w510]
            tunnel: w491 -> [_ w496 w512]
            frame "MM3000", Default {
            }
            frame "NI 735x" {
              n201 = disable-structure shown="Disabled" {
                disable-tunnel: w499 -> [w504 _]
                disable-tunnel: [w503 _] -> w498
                disable-tunnel: w497 -> [w502 _]
                disable-tunnel: w496 -> [w501 _]
                frame Disabled {
                  n202 = Unbundle By Name(w501) -> ("Motion Bd ID"=w500:u8)
                  n203 = call <vilib>:"Stop Program.flx"("error in (no error)"=w502, "Program (1)"=w504, "Board ID"=w500) -> ("error out"=w503:errorcluster)  [unwired: 3 in, 2 out]
                }
                frame Enabled {
                }
              }
            }
            frame "Galil" {
              n204 = Unbundle By Name(w512) -> ("GL Ref Out"=w506:refnum<k7>, "# Axis"=w511:i8)
              n205 = for {
                N: w511 -> [_]
                tunnel: [w516] -> w508
                tunnel: w506 -> [w515]
                tunnel: w510 -> [w513]
                i -> [w514]
                n206 = call "GL CheckForMotion.vi"("error in"=w513, "Axis"=w514, "Refnum in"=w515) -> ("error out"=w516:errorcluster)  [unwired: 6 in, 2 out]
              }
              n207 = call "GL Command Set.vi"("Command"=Command_Menu."Halt Execute", "error in (no error)"=w508, "Value"=-1, "Galil.IGalil"=w506) -> ("error out"=w507:errorcluster)  [unwired: 3 in, 4 out]
            }
          }
        }
      }
      n208 = Index Array(array=w463) -> (element=w462:T17)  [unwired: 1 in]
      n209 = Unbundle By Name(w441) -> ("status"=w455:bool)
      n210 = Unbundle By Name(w462) -> ("gain"=w461:dbl)
    }
    frame "LeCroy" {
      w611 = u16 0 items=["Channel 1", "Channel 2", "Channel 3", "Channel 4", "Memory 1", "Memory 2", "Memory 3", "Memory 4", "Function 1", "Function 2", "Function 3", "Function 4", "Function 5", "Function 6", "Function 7", "Function 8", "Other"] ("Source (0: Channel 1)")
      # "Set flip flop to take next frame edge"
      # "Arm digitizer"
      n211 = Unbundle By Name(w613) -> ("Digitizer ID Cluster.LeCroy VISA"=w615:refnum<visa-resource-name>)
      n212 = call <instrlib>:"Initiate.vi"("error in (no error)"=w614, "VISA resource name"=w615) -> ("error out"=w616:errorcluster)  [unwired: 8 in, 1 out]
      n213 = Unbundle By Name(w599) -> ("Motion System"=w621:T3)
      n214 = case shown="True" w620 {
        tunnel: w616 -> [w679 w685]
        tunnel: [w679 w684] -> w603
        tunnel: w622 -> [_ w683]
        tunnel: [u8 0 ("Resource Out") w682] -> w625
        tunnel: w621 -> [_ w681]
        tunnel: w599 -> [_ w680]
        frame False {
        }
        frame True {
          n215 = case shown="\"Galil\"" w681 {
            tunnel: w685 -> [w686 w691 _]
            tunnel: [w686 w690 w706] -> w684
            tunnel: w683 -> [_ w689 w702]
            tunnel: [_ w687 _] -> w682
            tunnel: w680 -> [_ w688 w705]
            frame "MM3000", Default {
            }
            frame "NI 735x" {
              n216 = disable-structure shown="Disabled" {
                disable-tunnel: w691 -> [w700 _]
                disable-tunnel: [w699 _] -> w690
                disable-tunnel: w689 -> [w695 _]
                disable-tunnel: w688 -> [w694 _]
                disable-tunnel: [w692 _] -> w687
                frame Disabled {
                  n217 = Unbundle By Name(w694) -> ("Motion Bd ID"=w693:u8)
                  n218 = Select(t=T12 6 ("Motion Program"), s=w695, f=T12 7 ("Motion Program")) -> (s? t:f=w696:T12)
                  n219 = call <vilib>:"Run Program.flx"("error in (no error)"=w700, "Program (1)"=w696, "Board ID"=w693) -> ("error out"=w699:errorcluster, "Resource Out"=w692:T14)  [unwired: 3 in, 1 out]
                }
                frame Enabled {
                }
              }
            }
            frame "Galil" {
              n220 = Unbundle By Name(w705) -> ("GL Ref Out"=w710:refnum<k7>)
              n221 = Select(t="#FORMOD" ("Program Name"), s=w702, f="#BACKMOD" ("Program Name")) -> (s? t:f=w709:string)
              n222 = Select(t=u8 6 ("Motion Program"), s=w702, f=u8 7 ("Motion Program")) -> (s? t:f=w703:u8)
              n223 = call "GL Command Set.vi"("Command"=Command_Menu."Execute", "Text Input"=w709, "Value"=w703, "Galil.IGalil"=w710) -> ("error out"=w706:errorcluster)  [unwired: 3 in, 4 out]
            }
          }
        }
      }
      n224 = Unbundle By Name(w599) -> ("Motion System"=w600:T3)
      n225 = case shown="\"Galil\"" w600 {
        tunnel: w601 -> [_ w638]
        tunnel: w599 -> [w632 _]
        tunnel: w603 -> [w631 w637]
        tunnel: [w630 w636] -> w602
        frame "Galil" {
          n226 = Unbundle By Name(w632) -> ("GL Ref Out"=w635:refnum<k7>)
          n227 = call "GL Command Set.vi"("Command"=Command_Menu."Set Bit", "error in (no error)"=w631, "Value"=19, "Galil.IGalil"=w635) -> ("error out"=w630:errorcluster)  [unwired: 3 in, 4 out]
        }
        frame "NI 735x", Default {
          n228 = call-poly <vilib>:"DAQmx Write.vi"("task/channels in"=w638, "data"=TRUE ("stop (T)"), "error in"=w637) -> ("error out"=w636:errorcluster)  [unwired: 10 in, 2 out]
        }
      }
      n229 = Unbundle By Name(w599) -> ("Motion System"=w604:T3)
      n230 = case shown="True" FALSE {
        tunnel: w602 -> [w713 w717]
        tunnel: [w713 w716] -> w617
        tunnel: w599 -> [_ w715]
        tunnel: w604 -> [_ w714]
        frame False {
          n231 = Wait (ms)(milliseconds to wait=u32 50) -> ()  [unwired: 1 out]
        }
        frame True {
          n232 = case shown="\"NI 735x\"" w714 {
            tunnel: w717 -> [w718 w722]
            tunnel: [w718 w721] -> w716
            tunnel: w715 -> [_ w720]
            frame "MM3000", Default {
            }
            frame "NI 735x" {
              n233 = Unbundle By Name(w720) -> ("Motion Bd ID"=w719:u8)
              n234 = call "CheckPause.vi"("error in"=w722, "Motion Board ID"=w719) -> ("error out"=w721:errorcluster)  [unwired: 3 in]
            }
          }
        }
      }
      n235 = Unbundle By Name(w613) -> ("Dig Ch"=w628:i32)  [unwired: 1 out]
      n236 = case shown="\"NI 735x\", Default" w604 {
        tunnel: w617 -> [w743 w751 w759]
        tunnel: [w742 w751 w759] -> w610
        tunnel: [w741 -5 ("Output") w753] -> w618
        tunnel: w599 -> [w740 _ w758]
        frame "NI 735x", Default {
          n237 = disable-structure shown="Disabled" {
            disable-tunnel: w743 -> [w748 _]
            disable-tunnel: [w747 _] -> w742
            disable-tunnel: [w746 _] -> w741
            disable-tunnel: w740 -> [w745 _]
            frame Disabled {
              n238 = Unbundle By Name(w745) -> ("Motion Bd ID"=w744:u8)
              n239 = call <vilib>:"Read Variable.flx"("Var"=T13 4, "error in (no error)"=w748, "Board ID"=w744) -> ("error out"=w747:errorcluster, "Output"=w746:i32)  [unwired: 1 in, 4 out]
            }
            frame Enabled {
            }
          }
        }
        frame "No Motion Card" {
        }
        frame "Galil" {
          (unwired) -5 ("Output")
          n240 = Unbundle By Name(w758) -> ("GL Ref Out"=w757:refnum<k7>, "scan pair"=w755:T4)
          n241 = call "GetScanAxis.vi"("scan pair"=w755) -> ("Axis 1"=w754:i32)  [unwired: 1 in, 2 out]
          n242 = Decrement(x=w754) -> (x-1=w752:i32)
          n243 = call "GL Command Set.vi"("Command"=Command_Menu."Tell Velocity", "Axis"=w752, "Galil.IGalil"=w757) -> ("Response#"=w753:i32)  [unwired: 4 in, 4 out]
        }
      }
      n244 = Number To Decimal String(number=w628) -> ()  [unwired: 1 in, 1 out]
      n245 = call "GetAcqSeqLeCroy.vi"("Digitizer Settings"=w613, "errorin"=w610, "Source (0: Channel 1)"=w611, "save?"=FALSE) -> ("Raw VGain (scale)"=w607:dbl, "Data Array"=w609:i16[][], "error out"=w608:errorcluster)  [unwired: 17 in, 4 out]
      n246 = case shown="\"NI 735x\", Default" w604 {
        tunnel: w608 -> [w725 w735 w739]
        tunnel: [w724 w734 w739] -> w605
        tunnel: w599 -> [w723 w737 _]
        frame "NI 735x", Default {
          n247 = disable-structure shown="Disabled" {
            disable-tunnel: w725 -> [w729 _]
            disable-tunnel: [w728 _] -> w724
            disable-tunnel: w723 -> [w727 _]
            frame Disabled {
              n248 = Unbundle By Name(w727) -> ("Motion Bd ID"=w726:u8)
              n249 = call <vilib>:"Read Variable.flx"("Var"=T13 4, "error in (no error)"=w729, "Board ID"=w726) -> ("error out"=w728:errorcluster)  [unwired: 1 in, 5 out]
            }
            frame Enabled {
            }
          }
        }
        frame "Galil" {
          n250 = Unbundle By Name(w737) -> ("GL Ref Out"=w736:refnum<k7>, "scan pair"=w733:T4)
          n251 = call "GetScanAxis.vi"("scan pair"=w733) -> ("Axis 1"=w732:i32)  [unwired: 1 in, 2 out]
          n252 = Decrement(x=w732) -> (x-1=w731:i32)
          n253 = call "GL Command Set.vi"("Command"=Command_Menu."Tell Velocity", "error in (no error)"=w735, "Axis"=w731, "Galil.IGalil"=w736) -> ("error out"=w734:errorcluster)  [unwired: 3 in, 4 out]
        }
        frame "No Motion Card" {
        }
      }
      n254 = case shown="\"NI 735x\", Default" w604 {
        tunnel: w601 -> [_ w648]
        tunnel: w599 -> [w640 _]
        tunnel: w605 -> [w642 w647]
        tunnel: [w641 w646] -> w606
        frame "Galil" {
          n255 = Unbundle By Name(w640) -> ("GL Ref Out"=w645:refnum<k7>)
          n256 = call "GL Command Set.vi"("Command"=Command_Menu."Clear Bit", "error in (no error)"=w642, "Value"=19, "Galil.IGalil"=w645) -> ("error out"=w641:errorcluster)  [unwired: 3 in, 4 out]
        }
        frame "NI 735x", Default {
          n257 = call-poly <vilib>:"DAQmx Write.vi"("task/channels in"=w648, "data"=FALSE ("stop (T)"), "error in"=w647) -> ("error out"=w646:errorcluster)  [unwired: 10 in, 2 out]
        }
      }
      n258 = Less Than 0?(x=w618) -> (x < 0?=w627:bool)
      n259 = Not(x=w627) -> (.not. x?=w623:bool)
      n260 = case shown="True" w620 {
        tunnel: w625 -> [_ w655]
        tunnel: w606 -> [w650 w653]
        tunnel: [w650 w654] -> w619
        tunnel: w599 -> [_ w652]
        frame False {
        }
        frame True {
          n261 = Unbundle By Name(w652) -> ("Motion System"=w651:T3)
          n262 = case shown="\"NI 735x\"" w651 {
            tunnel: w655 -> [_ w660 _]
            tunnel: [w656 w659 w668] -> w654
            tunnel: w653 -> [w656 w658 w671]
            tunnel: w652 -> [_ w657 w673]
            frame "MM3000", Default {
            }
            frame "NI 735x" {
              n263 = disable-structure shown="Disabled" {
                disable-tunnel: w660 -> [w665 _]
                disable-tunnel: [w664 _] -> w659
                disable-tunnel: w658 -> [w663 _]
                disable-tunnel: w657 -> [w662 _]
                frame Disabled {
                  n264 = Unbundle By Name(w662) -> ("Motion Bd ID"=w661:u8)
                  n265 = call <vilib>:"Stop Program.flx"("error in (no error)"=w663, "Program (1)"=w665, "Board ID"=w661) -> ("error out"=w664:errorcluster)  [unwired: 3 in, 2 out]
                }
                frame Enabled {
                }
              }
            }
            frame "Galil" {
              n266 = Unbundle By Name(w673) -> ("GL Ref Out"=w667:refnum<k7>, "# Axis"=w672:i8)
              n267 = for {
                N: w672 -> [_]
                tunnel: [w677] -> w669
                tunnel: w667 -> [w676]
                tunnel: w671 -> [w674]
                i -> [w675]
                n268 = call "GL CheckForMotion.vi"("error in"=w674, "Axis"=w675, "Refnum in"=w676) -> ("error out"=w677:errorcluster)  [unwired: 6 in, 2 out]
              }
              n269 = call "GL Command Set.vi"("Command"=Command_Menu."Halt Execute", "error in (no error)"=w669, "Value"=-1, "Galil.IGalil"=w667) -> ("error out"=w668:errorcluster)  [unwired: 3 in, 4 out]
            }
          }
        }
      }
      n270 = Select(t=w623, s=w620, f=w622) -> (s? t:f=w626:bool)
      n271 = Unbundle By Name(w619) -> ("status"=w629:bool)
    }
    frame "AlazarTech" {
      # "Set flip flop to take next frame edge"
      n272 = Unbundle By Name(w760) -> ("Motion System"=w765:T3)
      n273 = Unbundle By Name(w768) -> ("Digitizer ID Cluster.Acqiris/Alazar/SP ID"=w786:u32[])
      n274 = case shown="\"NI 735x\", Default" w765 {
        tunnel: w762 -> [_ w809]
        tunnel: w760 -> [w803 _]
        tunnel: w766 -> [w802 w807]
        tunnel: [w801 w808] -> w767
        frame "Galil" {
          n275 = Unbundle By Name(w803) -> ("GL Ref Out"=w806:refnum<k7>)
          n276 = call "GL Command Set.vi"("Command"=Command_Menu."Set Bit", "error in (no error)"=w802, "Value"=19, "Galil.IGalil"=w806) -> ("error out"=w801:errorcluster)  [unwired: 3 in, 4 out]
        }
        frame "NI 735x", Default {
          n277 = call-poly <vilib>:"DAQmx Write.vi"("task/channels in"=w809, "data"=TRUE ("stop (T)"), "error in"=w807) -> ("error out"=w808:errorcluster)  [unwired: 10 in, 2 out]
        }
      }
      n278 = Index Array(array=w786) -> (element=w779:u32)  [unwired: 1 in]
      n279 = call "Rapid Read_Alazar_Done - ATS-SDK.vi"("Handle"=w779, "Motion Settings"=w760, "error out"=w767, "Pause?"=w773) -> ("Handle Out"=w778:u32, "Reverse?"=w776:bool, "error out"=w775:errorcluster)  [unwired: 9 in]
      n280 = case shown="14" 0 ("lines per plane") {
        tunnel: [_ u16 3 ("Extra Shift")] -> w781
        frame 0, Default {
        }
        frame 14 {
        }
      }
      n281 = expression code="x*1000"(w774) -> (w780:sgl)
      n282 = Unbundle By Name(w768) -> ("lines per plane"=w770:i32, "rf points per line"=w769:i32)
      n283 = call "AlazarReadBuffer - ATS-SDK.vi"("Handle"=w778, "Digitizer Settings"=w768, "time out (ms)"=w780, "AlazarCluster"="AlazarCluster", "Extra Shift"=w781, "error in (no error)"=w775) -> ("Data Array"=w772:i16[], "Return Code"=w783:u32, "Voltage Scale"=w785:dbl, "error out"=w764:errorcluster)  [unwired: 5 in, 1 out]
      n284 = Unbundle By Name("AlazarCluster") -> ("rf pts actual"=w790:u32)
      n285 = Equal?(x=w783, y=u32 579) -> (x = y?=w782:bool)
      n286 = call "DelayPtsAdjust.vi"("Digitizer Settings"=w768) -> ("PostDelayCorrection"=w771:u32)  [unwired: 9 in, 1 out]
      n287 = Reshape Array(w772, w770, w790) -> (w788:i16[][])
      n288 = Array Subset(array=w788, index (col)=w771, length (col)=w769) -> (w789:i16[][])  [unwired: 2 in]
      n289 = Unbundle By Name(w760) -> ("Motion System"=w761:T3)
      n290 = case shown="\"NI 735x\", Default" w761 {
        tunnel: w762 -> [_ w799]
        tunnel: w760 -> [w793 _]
        tunnel: w764 -> [w792 w797]
        tunnel: [w791 w798] -> w763
        frame "Galil" {
          n291 = Unbundle By Name(w793) -> ("GL Ref Out"=w796:refnum<k7>)
          n292 = call "GL Command Set.vi"("Command"=Command_Menu."Clear Bit", "error in (no error)"=w792, "Value"=19, "Galil.IGalil"=w796) -> ("error out"=w791:errorcluster)  [unwired: 3 in, 4 out]
        }
        frame "NI 735x", Default {
          n293 = call-poly <vilib>:"DAQmx Write.vi"("task/channels in"=w799, "data"=FALSE ("stop (T)"), "error in"=w797) -> ("error out"=w798:errorcluster)  [unwired: 10 in, 2 out]
        }
      }
    }
  }
  "Array" <- w16
  "error out" <- w18
  "gain" <- w15
  "dig error" <- w13
  n294 = case shown="\"Stony Brook\"" "Location" {
    tunnel: w5 -> [w812 w814]
    tunnel: [w812 w813] -> w4
    frame "WCM Main", Default {
    }
    frame "Stony Brook" {
      n295 = Not(x=w814) -> (.not. x?=w813:bool)
    }
  }
  "Reverse?" <- w4
